vi "Add Sequence Error Message.vi"(8 "error in (no error)":errorcluster, 9 "Msg":string, 10 "Seq Path":string, 11 "Variant in":variant) -> (0 "error out":errorcluster, 3 "Variant out":variant)   [LabVIEW 2016, in "SLL TestStand.lvlib"]
uses:
  SLL TestStand.lvlib
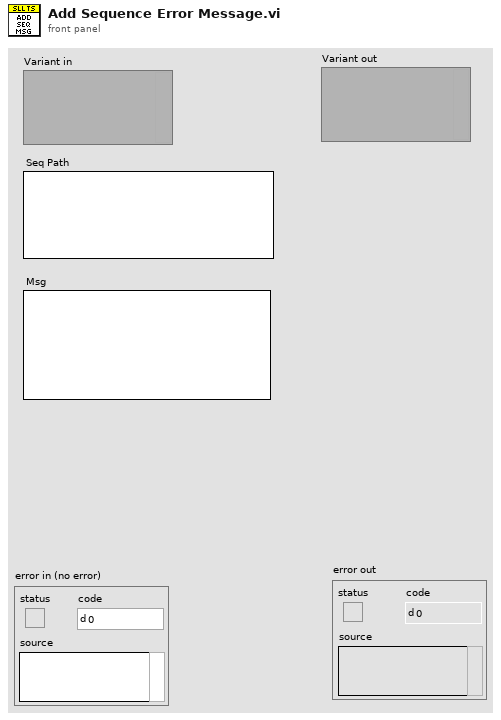
[diagram p1: front panel]
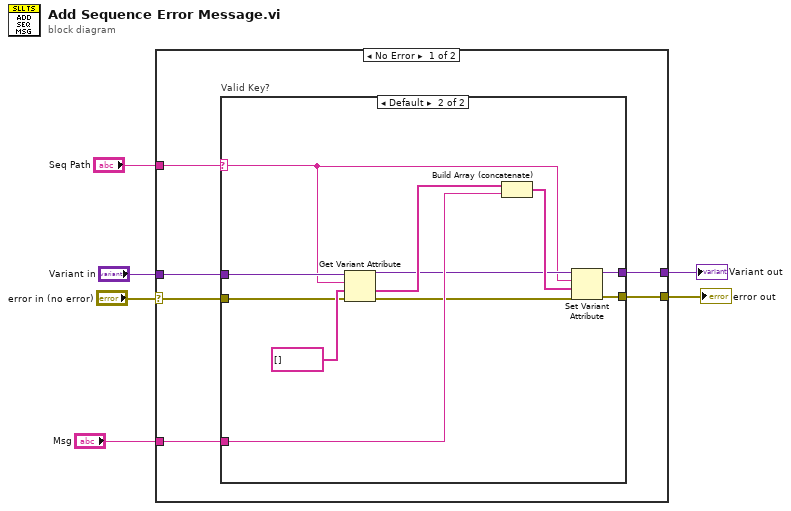
[diagram p0: block diagram]
diagram:
  n1 = case shown="No Error" "error in (no error)" {
    selector: "error in (no error)" -> [w9 w27]
    tunnel: [w12 w26] -> w6
    tunnel: "Msg" -> [w11 _]
    tunnel: "Variant in" -> [w10 w26]
    tunnel: [w8 w27] -> w2
    tunnel: "Seq Path" -> [w7 _]
    frame No Error {
      n2 = case "Valid Key?" shown="Default" w7 {
        selector: w7 -> [_ w15]
        tunnel: [w14 w25] -> w12
        tunnel: w11 -> [_ w23]
        tunnel: w10 -> [w14 w19]
        tunnel: w9 -> [w13 w18]
        tunnel: [w13 w17] -> w8
        frame "" {
          # "No Key. Ignore"
        }
        frame Default {
          n3 = Get Variant Attribute(Variant=w19, name=w15, default value (empty Variant)=string[] [], error in=w18) -> (duplicate Variant=w21:variant, value=w22:string[], error out=w16:errorcluster)  [unwired: 1 out]
          n4 = Build Array (concatenate)(w22, w23) -> (w24:string[])
          n5 = Set Variant Attribute(Variant=w21, name=w15, value=w24, error in=w16) -> (Variant out=w25:variant, error out=w17:errorcluster)  [unwired: 1 out]
        }
      }
    }
    frame Error {
    }
  }
  "Variant out" <- w6
  "error out" <- w2
